vi "Meas Proc QWTB Generate Algorithm Info Section.vi"(7 "processing setup":T1={"mode"=enum."Raw", "call after avgs?"=FALSE, "calculate?"=FALSE, "raw mode"={"command"="", "result mode"=enum."Display console output (only Octave)", "res variable"=""}, "QWTB"={"QWTB path"=path "", "alg filter path"="", "alg ids"=[], "alg parameters"=[], "parsed parameters"=[], "selected alg id"="", "selected unc mode"=enum."None", "qwtb mcc"=100, "qwtb timeout"=90, "qwtb covg"=95.0, "qwtb ofs"=0, "qwtb lim data"=0, "multicore"={"jobs folder"=path "", "cores"=0, "max jobs"=0, "mode"=enum."Singlecore"}, "unc once?"=FALSE, "qwtb tstemp"=enum."Enabled (default)", "octave reset"=FALSE, "exec mode"=enum."Single-core"}}, 8 "sections in":string[](array[string]), 10 "sequence item":T12, 11 "new info data in":string) -> (0 "sections out":string[](array[string]), 3 "new info data out":string)   [LabVIEW 2020]
doc: "This VI will write QWTB calculation data into the measurement info header."
uses:
  Meas Sequence Item.ctl
  Meas Sampling Configuration.ctl
  adc/ADC Trig Config.ctl
  adc/ADC Trig Mode Source.ctl
  adc/ADC Trig Slope.ctl
  adc/ADC Trig Coupling.ctl
  Meas Proc QWTB Algorithm Parameter Data.ctl
  drivers/DMM/3458A Sampling Rate.ctl
  drivers/AWG/AWG Clock Setup Mode.ctl
  Meas Process Config.ctl
  Meas Process Mode.ctl
  Meas Process Raw Config.ctl
  Meas Process Raw Result Mode.ctl
  Meas Proc QWTB Setup.ctl
  Meas Proc QWTB Uncertainty Mode.ctl
  Meas Proc QWTB Multicore Setup.ctl
  Meas Proc QWTB Multicore Type.ctl
  Meas Process Time Stamp Mode.ctl
  Meas Proc QWTB Exec Mode.ctl
  octave/infolib/String.vi
  octave/infolib/Boolean.vi
  octave/infolib/I64.vi
  octave/infolib/EXT.vi
  octave/infolib/1D String.vi
  octave/infolib/infolib.lvlib
  drivers/AWG/AWG.lvlib
  drivers/DMM/3458A Virtual Digitizer.lvlib
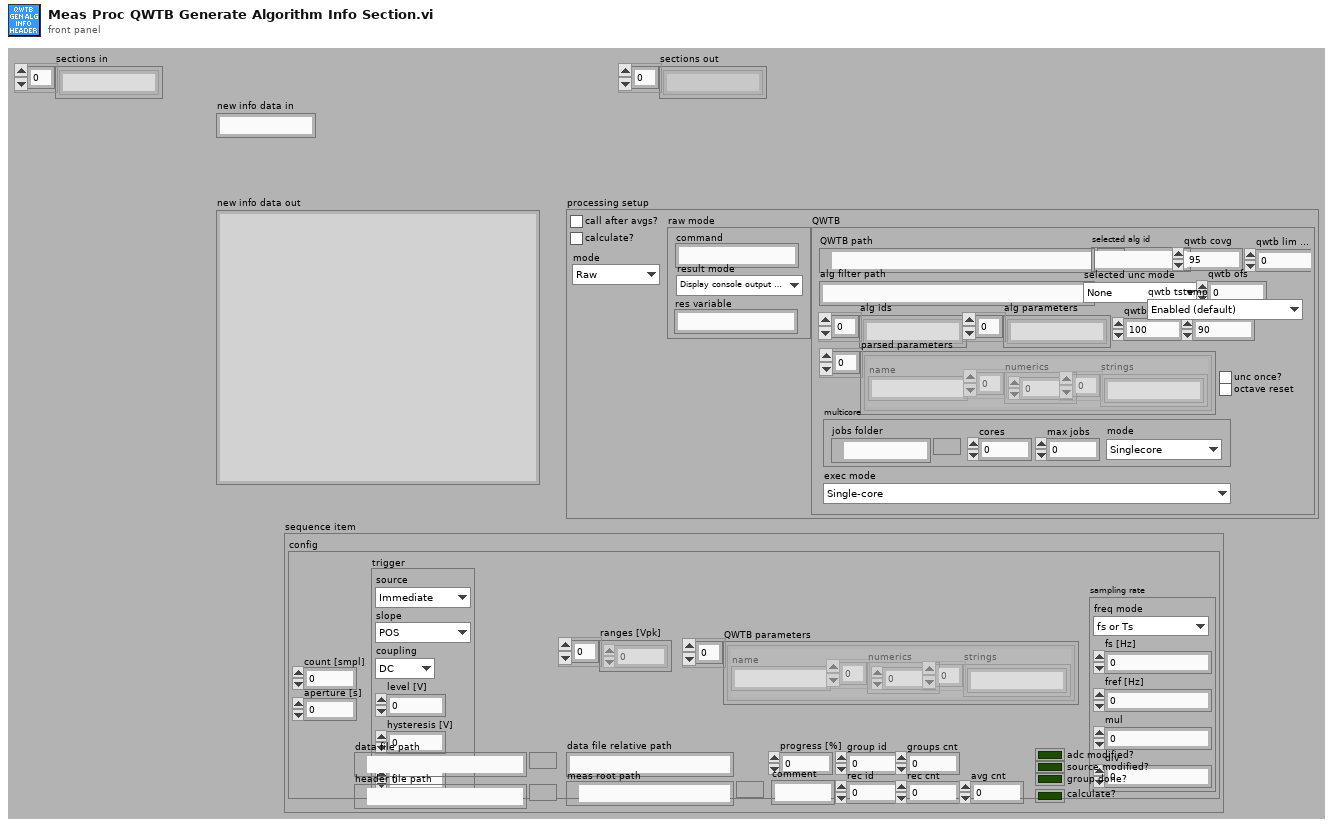
[diagram p1: front panel]
types:
  T1 = typedef "Meas Process Config.ctl" = cluster{"mode":T2, "call after avgs?":bool, "calculate?":bool, "raw mode":T3, "QWTB":T5}
  T2 = typedef "Meas Process Mode.ctl" = enum16{"Raw", "QWTB"}
  T3 = typedef "Meas Process Raw Config.ctl" = cluster{"command":string, "result mode":T4, "res variable":string}
  T4 = typedef "Meas Process Raw Result Mode.ctl" = enum16{"Display console output (only Octave)", "Display string variable", "Display result file %respath%"}
  T5 = typedef "Meas Proc QWTB Setup.ctl" = cluster{"QWTB path":path, "alg filter path":string, "alg ids":string[], "alg parameters":string[], "parsed parameters":T6[], "selected alg id":string, "selected unc mode":T7, "qwtb mcc":i32, "qwtb timeout":i32, "qwtb covg":dbl, "qwtb ofs":i64, "qwtb lim data":i64, "multicore":T8, "unc once?":bool, "qwtb tstemp":T10, "octave reset":bool, "exec mode":T11}
  T6 = typedef "Meas Proc QWTB Algorithm Parameter Data.ctl" = cluster{"name":string, "numerics":dbl[], "strings":string[]}
  T7 = typedef "Meas Proc QWTB Uncertainty Mode.ctl" = enum16{"None", "GUF", "Monte Carlo"}
  T8 = typedef "Meas Proc QWTB Multicore Setup.ctl" = cluster{"jobs folder":path, "cores":i32, "max jobs":i32, "mode":T9}
  T9 = typedef "Meas Proc QWTB Multicore Type.ctl" = enum16{"Singlecore", "Multicore", "Multistation"}
  T10 = typedef "Meas Process Time Stamp Mode.ctl" = enum16{"Enabled (default)", "Disabled", "Relative to 1. record"}
  T11 = typedef "Meas Proc QWTB Exec Mode.ctl" = enum16{"Single-core", "Parallel Record Processing"}
  T12 = typedef "Meas Sequence Item.ctl" = cluster{"config":T13, "data file path":path, "header file path":path, "group id":i32, "rec id":i32, "group done?":bool, "adc modified?":bool, "source modified?":bool, "progress [%]":dbl, "groups cnt":i32, "rec cnt":i32, "data file relative path":string, "meas root path":path, "calculate?":bool, "comment":string, "avg cnt":i32}
  T13 = typedef "Meas Sampling Configuration.ctl" = cluster{"count [smpl]":i64, "aperture [s]":dbl, "trigger":T14, "ranges [Vpk]":dbl[], "QWTB parameters":T6[], "sampling rate":T18}
  T14 = typedef "ADC Trig Config.ctl" = cluster{"source":T15, "slope":T16, "coupling":T17, "level [V]":dbl, "hysteresis [V]":dbl, "pre-trigger [%]":dbl}
  T15 = typedef "ADC Trig Mode Source.ctl" = enum16{"Immediate", "External", "Level"}
  T16 = typedef "ADC Trig Slope.ctl" = enum16{"POS", "NEG"}
  T17 = typedef "ADC Trig Coupling.ctl" = enum16{"DC", "AC"}
  T18 = typedef "3458A Virtual Digitizer.lvlib/3458A Sampling Rate.ctl" = cluster{"freq mode":T19, "fs [Hz]":dbl, "fref [Hz]":dbl, "mul":dbl, "div":dbl}
  T19 = typedef "AWG.lvlib/AWG Clock Setup Mode.ctl" = enum16{"fs or Ts", "fs or Ts with fref", "fref/N", "fref*M/N", "fref*Ratio"}
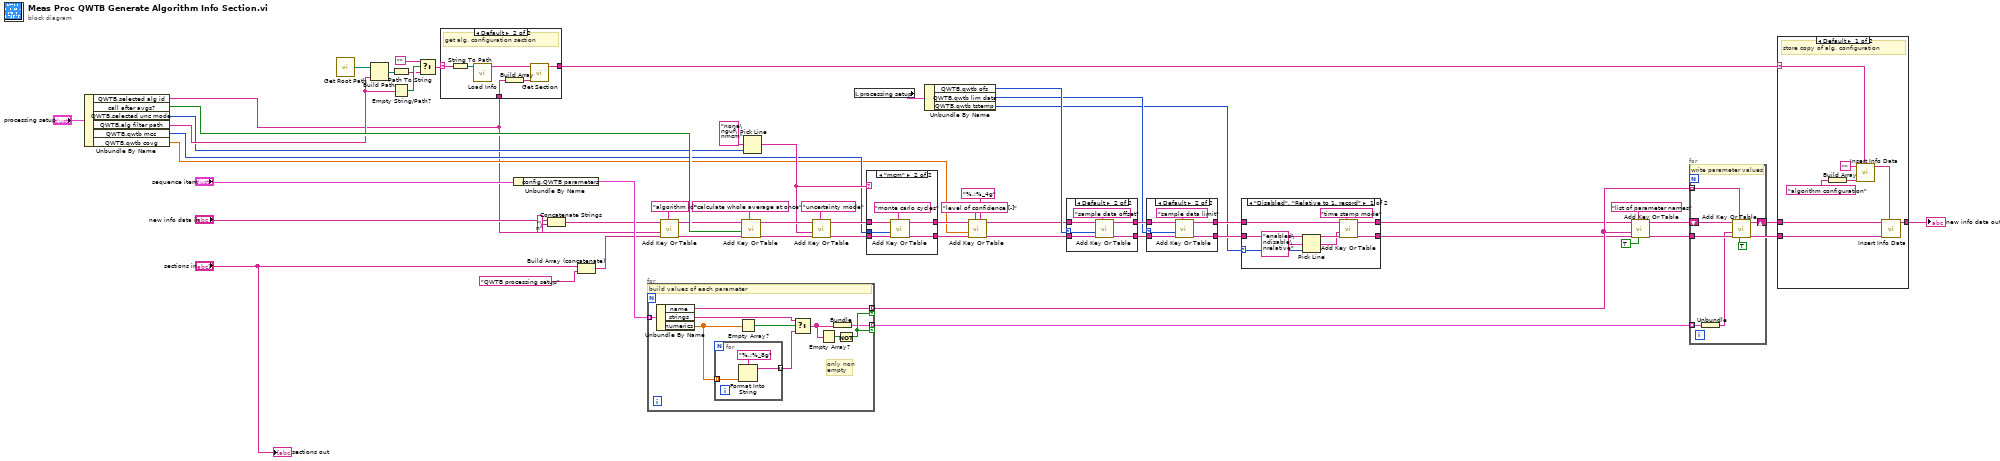
[diagram p0: block diagram]
diagram:
  n1 = Unbundle By Name("processing setup") -> ("QWTB.selected alg id"=w14:string, "call after avgs?"=w53:bool, "QWTB.selected unc mode"=w25:T7, "QWTB.alg filter path"=w52:string, "QWTB.qwtb mcc"=w20:i32, "QWTB.qwtb covg"=w16:dbl)
  n2 = call "Get Root Path.vi"() -> ("root path"=w26:path)
  n3 = Build Path(base path=w26, name or relative path=w52) -> (appended path=w38:path)
  n4 = Path To String(path=w38) -> (string=w27:string)
  n5 = Empty String/Path?(string/path=w52) -> (empty?=w37:bool)
  n6 = Select(t="", s=w37, f=w27) -> (s? t:f=w28:string)
  n7 = case shown="Default" w28 {
    selector: w28 -> [_ w63]
    tunnel: w14 -> [_ w61]
    tunnel: [_ w60] -> w29
    frame "" {
    }
    frame Default {
      # "get alg. configuration section"
      n8 = String To Path(string=w63) -> (path=w62:path)
      n9 = call "Load Info.vi"("filename"=w62) -> ("info data"=w59:string)  [unwired: 9 in, 1 out]
      n10 = Build Array(w61) -> (w58:string[])
      n11 = call "Get Section.vi"("sections"=w58, "info data"=w59) -> ("section part"=w60:string)  [unwired: 7 in, 2 out]
    }
  }
  n12 = Unbundle By Name("sequence item") -> ("config.QWTB parameters"=w48:T6[])
  n13 = Concatenate Strings("new info data in", "\n" ("string")) -> (w42:string)
  n14 = Build Array (concatenate)("sections in", "QWTB processing setup" ("section name")) -> (w43:string[])
  n15 = for {
    tunnel: w48 -> [w73] mode=indexing
    tunnel: [w72] -> w31 mode=indexing if=w66
    tunnel: [w64] -> w33 mode=indexing if=w66
    # "only non\nempty"
    # "build values of each parameter"
    n16 = Unbundle By Name(w73) -> ("name"=w72:string, "strings"=w69:string[], "numerics"=w71:dbl[])
    n17 = for {
      tunnel: w71 -> [w75] mode=indexing
      tunnel: [w74] -> w68 mode=indexing
      n18 = Format Into String(format string="%.;%_8g", w75) -> (resulting string=w74:string)  [unwired: 2 in, 1 out]
    }
    n19 = Empty Array?(array=w71) -> (empty?=w70:bool)
    n20 = Select(t=w69, s=w70, f=w68) -> (s? t:f=w65:string[])
    n21 = Empty Array?(array=w65) -> (empty?=w67:bool)
    n22 = Bundle("strings"=w65) -> (w64:cluster{"strings":string[]})  [unwired: 1 in]
    n23 = Not(x=w67) -> (.not. x?=w66:bool)
  }
  n24 = call-poly "Add Key Or Table.vi"("key description"="algorithm id", "sections"=w43, "string"=w14, "info data"=w42) -> ("sections out"=w45:string[], "info data out"=w44:string)  [unwired: 6 in]
  n25 = call-poly "Add Key Or Table.vi"("key description"="calculate whole average at once", "sections"=w45, "boolean"=w53, "info data"=w44) -> ("sections out"=w41:string[], "info data out"=w40:string)  [unwired: 6 in]
  n26 = Pick Line(multi-line string="none\nguf\nmcm", line index=w25) -> (output string=w21:string)  [unwired: 1 in]
  n27 = call-poly "Add Key Or Table.vi"("key description"="uncertainty mode", "sections"=w41, "string"=w21, "info data"=w40) -> ("sections out"=w22:string[], "info data out"=w23:string)  [unwired: 6 in]
  n28 = local read "processing setup"() -> (w13:T1)
  n29 = case shown="\"mcm\"" w21 {
    tunnel: w23 -> [w77 w84]
    tunnel: w22 -> [w78 w83]
    tunnel: [w78 w81] -> w17
    tunnel: [w77 w80] -> w18
    tunnel: w20 -> [_ w79]
    frame "False", Default {
    }
    frame "mcm" {
      n30 = call-poly "Add Key Or Table.vi"("key description"="monte carlo cycles", "sections"=w83, "numeric"=w79, "info data"=w84) -> ("sections out"=w81:string[], "info data out"=w80:string)  [unwired: 6 in]
    }
  }
  n31 = Unbundle By Name(w13) -> ("QWTB.qwtb ofs"=w12:i64, "QWTB.qwtb lim data"=w9:i64, "QWTB.qwtb tstemp"=w2:T10)
  n32 = call-poly "Add Key Or Table.vi"("format string (%.;%#_20f)"="%.;%_4g" ("format string (%_20f)"), "key description"="level of confidence [-]", "sections"=w17, "numeric"=w16, "info data"=w18) -> ("sections out"=w8:string[], "info data out"=w7:string)  [unwired: 5 in]
  n33 = case shown="Default" w12 {
    selector: w12 -> [_ w90]
    tunnel: w8 -> [w86 w92]
    tunnel: w7 -> [w85 w91]
    tunnel: [w86 w88] -> w11
    tunnel: [w85 w87] -> w10
    frame 0 {
    }
    frame Default {
      n34 = call-poly "Add Key Or Table.vi"("key description"="sample data offset", "sections"=w92, "numeric"=w90, "info data"=w91) -> ("sections out"=w88:string[], "info data out"=w87:string)  [unwired: 6 in]
    }
  }
  n35 = case shown="Default" w9 {
    selector: w9 -> [_ w98]
    tunnel: w11 -> [w94 w100]
    tunnel: w10 -> [w93 w99]
    tunnel: [w94 w96] -> w6
    tunnel: [w93 w95] -> w5
    frame 0 {
    }
    frame Default {
      n36 = call-poly "Add Key Or Table.vi"("key description"="sample data limit", "sections"=w100, "numeric"=w98, "info data"=w99) -> ("sections out"=w96:string[], "info data out"=w95:string)  [unwired: 6 in]
    }
  }
  n37 = case shown="\"Disabled\", \"Relative to 1. record\"" w2 {
    selector: w2 -> [w103 _]
    tunnel: w6 -> [w108 w110]
    tunnel: w5 -> [w107 w109]
    tunnel: [w105 w110] -> w4
    tunnel: [w104 w109] -> w3
    frame "Disabled", "Relative to 1. record" {
      n38 = Pick Line(multi-line string="enabled\ndisable\nrelative", line index=w103) -> (output string=w101:string)  [unwired: 1 in]
      n39 = call-poly "Add Key Or Table.vi"("key description"="time stamp mode", "sections"=w108, "string"=w101, "info data"=w107) -> ("sections out"=w105:string[], "info data out"=w104:string)  [unwired: 6 in]
    }
    frame Default {
    }
  }
  n40 = call-poly "Add Key Or Table.vi"("collumn vector (F)"=TRUE ("column vector (F)"), "key description"="list of parameter names", "sections"=w4, "string"=w31, "info data"=w3) -> ("sections out"=w34:string[], "info data out"=w32:string)  [unwired: 5 in]
  n41 = for {
    tunnel: w31 -> [w117] mode=indexing
    tunnel: w33 -> [w115] mode=indexing
    tunnel: w34 -> [w116]
    shift-right: [w113] -> w30
    shift-left: w32 -> [w112]
    # "write parameter values"
    n42 = Unbundle(w115) -> ("strings"=w114:string[])
    n43 = call-poly "Add Key Or Table.vi"("collumn vector (F)"=TRUE ("column vector (F)"), "key description"=w117, "sections"=w116, "string"=w114, "info data"=w112) -> ("info data out"=w113:string)  [unwired: 5 in, 1 out]
  }
  n44 = case shown="Default" w29 {
    selector: w29 -> [w122 _]
    tunnel: w34 -> [w121 _]
    tunnel: w30 -> [w118 w126]
    tunnel: [w125 w126] -> w57
    frame Default {
      # "store copy of alg. configuration"
      n45 = Build Array("algorithm configuration" ("section name")) -> (w123:string[])
      n46 = call "Insert Info Data.vi"("info data to insert"=w122, "sections"=w123, "info data"="") -> ("info data out"=w119:string)  [unwired: 7 in, 1 out]
      n47 = call "Insert Info Data.vi"("info data to insert"=w119, "sections"=w121, "info data"=w118) -> ("info data out"=w125:string)  [unwired: 7 in, 1 out]
    }
    frame "" {
    }
  }
  "new info data out" <- w57
  "sections out" <- "sections in"
